vi "fields save field.vi"(8 "error in (no error)":errorcluster, 9 "Post (empty)":T5, 10 "Field Id (\"\")":string, 11 "Connection Refnum":T4) -> (0 "error out":errorcluster, 1 "Field Record":T1={"ixField"=0, "iSequenceOrder"=0, "sxFieldId"="", "sxSequenceId"="", "sDisplayName"="", "sValue"="", "sUnits"="", "nDataType"=enum."timestamp", "nNextItem"=enum."Reset", "fSystem"=FALSE, "fSystemValue"=FALSE, "fRequired"=FALSE, "fSetAtTest"=FALSE, "fTestField"=FALSE, "fDeleted"=FALSE, "fIndexed"=FALSE, "fFreeList"=FALSE}, 3 "Connection Refnum":T4)   [LabVIEW 2011]
uses:
  Addons/internet/utils/keyedarr.llb/Keyed Array.ctl
  SI.LIB/ODBC/SQL Controls/Connection Refnum.ctl
  server/database/Fields/Field Record.ctl
  server/database/Fields/Field DataTypes.ctl
  server/database/Fields/Field NextItem.ctl
  Addons/internet/utils/strutil.llb/Case Matching.ctl
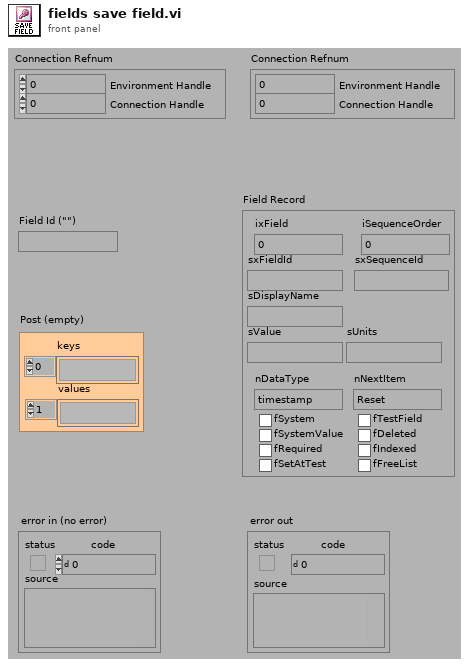
[diagram p1: front panel]
types:
  T1 = typedef "Field Record.ctl" = cluster{"ixField":i32, "iSequenceOrder":i32, "sxFieldId":string, "sxSequenceId":string, "sDisplayName":string, "sValue":string, "sUnits":string, "nDataType":T2, "nNextItem":T3, "fSystem":bool, "fSystemValue":bool, "fRequired":bool, "fSetAtTest":bool, "fTestField":bool, "fDeleted":bool, "fIndexed":bool, "fFreeList":bool}
  T2 = typedef "Field DataTypes.ctl" = enum32{"text", "numeric", "list", "timestamp", "boolean"}
  T3 = typedef "Field NextItem.ctl" = enum32{"Reset", "Retain", "Auto-Increment"}
  T4 = typedef "Connection Refnum.ctl" = cluster{"Environment Handle":i32, "Connection Handle":i32}
  T5 = typedef "Keyed Array.ctl" = cluster{"keys":string[], "values":string[]}
  T6 = typedef "Case Matching.ctl" = enum16{"a != A", "a == A", "system"}
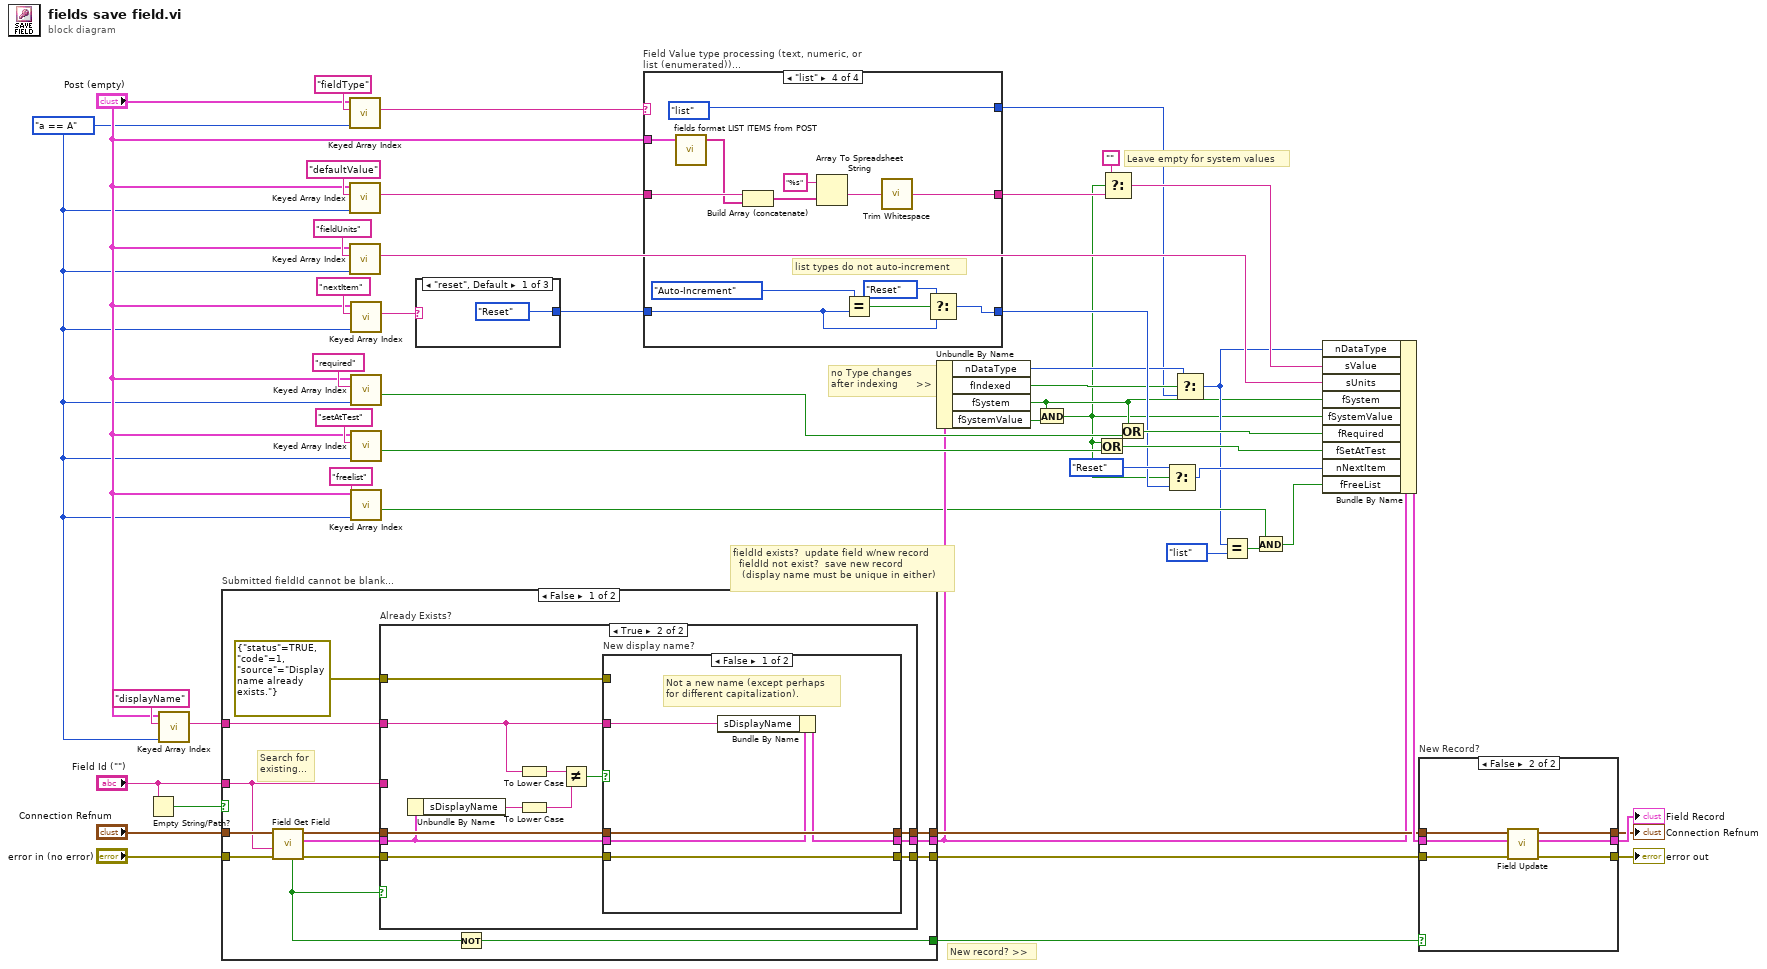
[diagram p0: block diagram]
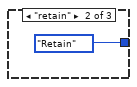
[diagram p2: hidden frame]
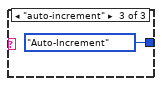
[diagram p3: hidden frame]
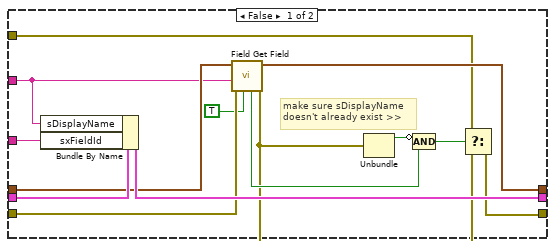
[diagram p4: hidden frame]
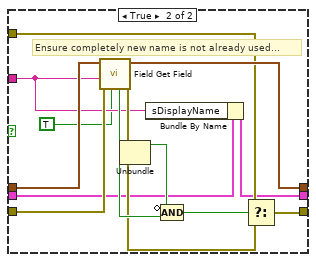
[diagram p5: hidden frame]
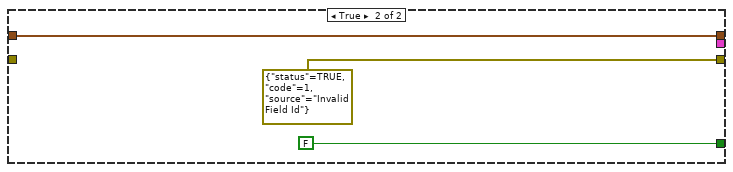
[diagram p6: hidden frame]
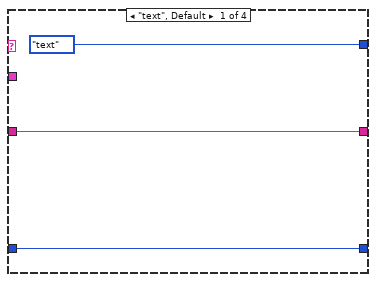
[diagram p7: hidden frame]
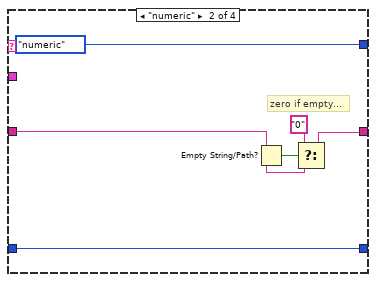
[diagram p8: hidden frame]
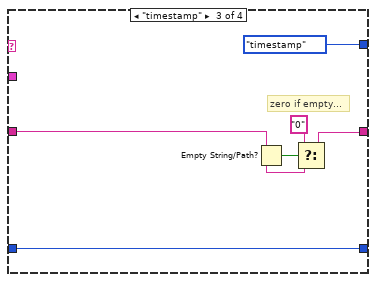
[diagram p9: hidden frame]
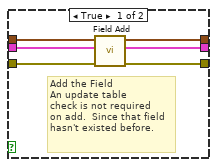
[diagram p10: hidden frame]
diagram:
  w14 = Case_Matching."a == A" ("case matching (sensitive)")
  # "no Type changes\nafter indexing      >>"
  # "Leave empty for system values"
  # "New record? >>"
  # "fieldId exists?  update field w/new record\n  fieldId not exist?  save new record\n   (display name must be unique in either)"
  n1 = Empty String/Path?(string/path="Field Id (\"\")") -> (empty?=w38:bool)
  n2 = call "Keyed Array Index.vi"("case matching (sensitive)"=w14, "key"="displayName", "array in"="Post (empty)") -> ("value"=w27:string)  [unwired: 1 in, 3 out]
  n3 = case "Submitted fieldId cannot be blank..." shown="False" w38 {
    tunnel: "Field Id (\"\")" -> [w52 _]
    tunnel: "Connection Refnum" -> [w62 w108]
    tunnel: "error in (no error)" -> [w61 _]
    tunnel: [w59 FALSE] -> w35
    tunnel: [w55 errorcluster {"status"=TRUE, "code"=1, "source"="Invalid Field Id"} ("error in (no error)")] -> w33
    tunnel: [w54 w108] -> w34
    tunnel: [w53 _] -> w12
    tunnel: w27 -> [w51 _]
    frame False {
      # "Search for\nexisting..."
      n4 = call "Field Get Field.vi"("error in (no error)"=w61, "sFieldId or sDisplayName (\"\")"=w52, "Connection Refnum"=w62) -> ("error out"=w58:errorcluster, "Field"=w56:T1, "Connection Refnum"=w57:T4, "Data Present?"=w60:bool)  [unwired: 2 in, 3 out]
      n5 = case "Already Exists?" shown="True" w60 {
        tunnel: w58 -> [w68 w85]
        tunnel: w57 -> [w70 w86]
        tunnel: w56 -> [w76 w82]
        tunnel: [w67 w84] -> w55
        tunnel: [w69 w83] -> w54
        tunnel: [w74 w81] -> w53
        tunnel: w52 -> [w75 _]
        tunnel: w51 -> [w64 w80]
        tunnel: errorcluster {"status"=TRUE, "code"=1, "source"="Display name already exists."} ("t") -> [w65 w79]
        frame False {
          # "make sure sDisplayName\ndoesn't already exist >>"
          n6 = Bundle By Name(cluster=w76, "sDisplayName"=w64, "sxFieldId"=w75) -> (w74:T1)
          n7 = call "Field Get Field.vi"("by sDisplayName? (f, by sFieldId)"=TRUE, "error in (no error)"=w68, "sFieldId or sDisplayName (\"\")"=w64, "Connection Refnum"=w70) -> ("error out"=w66:errorcluster, "Connection Refnum"=w69:T4, "Data Present?"=w72:bool)  [unwired: 1 in, 4 out]
          n8 = Unbundle(w66) -> ("status"=w73:bool)  [unwired: 2 out]
          n9 = Compound Arithmetic op=AND(invert w73, w72) -> (w71:bool)
          n10 = Select(t=w65, s=w71, f=w66) -> (s? t:f=w67:errorcluster)
        }
        frame True {
          n11 = Unbundle By Name(w82) -> ("sDisplayName"=w88:string)
          n12 = To Lower Case(string=w80) -> (all lower case string=w78:string)
          n13 = To Lower Case(string=w88) -> (all lower case string=w77:string)
          n14 = Not Equal?(x=w78, y=w77) -> (x != y?=w87:bool)
          n15 = case "New display name?" shown="False" w87 {
            tunnel: [w93 w104] -> w83
            tunnel: w86 -> [w93 w106]
            tunnel: [w92 w98] -> w84
            tunnel: w85 -> [w92 w105]
            tunnel: [w90 w95] -> w81
            tunnel: w82 -> [w91 w96]
            tunnel: w80 -> [w89 w97]
            tunnel: w79 -> [_ w99]
            frame False {
              # "Not a new name (except perhaps\nfor different capitalization)."
              n16 = Bundle By Name(cluster=w91, "sDisplayName"=w89) -> (w90:T1)
            }
            frame True {
              # "Ensure completely new name is not already used..."
              n17 = call "Field Get Field.vi"("by sDisplayName? (f, by sFieldId)"=TRUE, "error in (no error)"=w105, "sFieldId or sDisplayName (\"\")"=w97, "Connection Refnum"=w106) -> ("error out"=w100:errorcluster, "Connection Refnum"=w104:T4, "Data Present?"=w102:bool)  [unwired: 1 in, 4 out]
              n18 = Unbundle(w100) -> ("status"=w103:bool)  [unwired: 2 out]
              n19 = Bundle By Name(cluster=w96, "sDisplayName"=w97) -> (w95:T1)
              n20 = Compound Arithmetic op=AND(invert w103, w102) -> (w101:bool)
              n21 = Select(t=w99, s=w101, f=w100) -> (s? t:f=w98:errorcluster)
            }
          }
        }
      }
      n22 = Not(x=w60) -> (.not. x?=w59:bool)
    }
    frame True {
    }
  }
  n23 = call "Keyed Array Index.vi"("case matching (sensitive)"=w14, "key"="fieldType", "array in"="Post (empty)") -> ("value"=w43:string)  [unwired: 1 in, 3 out]
  n24 = call "Keyed Array Index.vi"("case matching (sensitive)"=w14, "key"="defaultValue", "array in"="Post (empty)") -> ("value"=w42:string)  [unwired: 1 in, 3 out]
  n25 = call "Keyed Array Index.vi"("case matching (sensitive)"=w14, "key"="fieldUnits", "array in"="Post (empty)") -> ("value"=w18:string)  [unwired: 1 in, 3 out]
  n26 = call "Keyed Array Index.vi"("case matching (sensitive)"=w14, "key"="nextItem", "array in"="Post (empty)") -> ("value"=w25:string)  [unwired: 1 in, 3 out]
  n27 = call "Keyed Array Index.vi"("case matching (sensitive)"=w14, "key"="required", "array in"="Post (empty)") -> ("valid key"=w31:bool)  [unwired: 1 in, 3 out]
  n28 = call "Keyed Array Index.vi"("case matching (sensitive)"=w14, "key"="setAtTest", "array in"="Post (empty)") -> ("valid key"=w29:bool)  [unwired: 1 in, 3 out]
  n29 = call "Keyed Array Index.vi"("case matching (sensitive)"=w14, "key"="freelist", "array in"="Post (empty)") -> ("valid key"=w10:bool)  [unwired: 1 in, 3 out]
  n30 = case shown="\"reset\", Default" w25 {
    tunnel: [Field_NextItem."Reset" ("nNextItem") Field_NextItem."Retain" ("nNextItem") Field_NextItem."Auto-Increment" ("nNextItem")] -> w24
    frame "reset", Default {
    }
    frame "retain" {
    }
    frame "auto-increment" {
    }
  }
  n31 = case "Field Value type processing (text, numeric, or list (enumerated))..." shown="\"list\"" w43 {
    tunnel: w42 -> [w114 w117 w123 w133]
    tunnel: "Post (empty)" -> [_ _ _ w137]
    tunnel: w24 -> [w115 w121 w127 w138]
    tunnel: [w115 w121 w127 w139] -> w13
    tunnel: [w114 w118 w124 w128] -> w21
    tunnel: [Field_DataTypes."text" ("x") Field_DataTypes."numeric" ("x") Field_DataTypes."timestamp" ("x") Field_DataTypes."list" ("x")] -> w5
    frame "text", Default {
    }
    frame "numeric" {
      # "zero if empty..."
      n32 = Empty String/Path?(string/path=w117) -> (empty?=w120:bool)
      n33 = Select(t="0", s=w120, f=w117) -> (s? t:f=w118:string)
    }
    frame "timestamp" {
      # "zero if empty..."
      n34 = Empty String/Path?(string/path=w123) -> (empty?=w126:bool)
      n35 = Select(t="0", s=w126, f=w123) -> (s? t:f=w124:string)
    }
    frame "list" {
      # "list types do not auto-increment"
      n36 = call "fields format LIST ITEMS from POST.vi"("Post (empty)"=w137) -> ("List Options"=w132:string[])  [unwired: 4 out]
      n37 = Build Array (concatenate)(w133, w132) -> (w131:string[])
      n38 = Array To Spreadsheet String(array=w131, 3:"%s" ("format string")) -> (spreadsheet string=w130:string)  [unwired: 1 out]
      n39 = Equal?(x=Field_NextItem."Auto-Increment" ("nNextItem"), y=w138) -> (x = y?=w140:bool)
      n40 = call <vilib>:"Trim Whitespace.vi"("string"=w130) -> ("trimmed string"=w128:string)  [unwired: 1 in]
      n41 = Select(t=Field_NextItem."Reset" ("nNextItem"), s=w140, f=w138) -> (s? t:f=w139:T3)
    }
  }
  n42 = Unbundle By Name(w12) -> ("nDataType"=w7:T2, "fIndexed"=w6:bool, "fSystem"=w2:bool, "fSystemValue"=w3:bool)
  n43 = And(x=w2, y=w3) -> (x .and. y?=w1:bool)
  n44 = Or(x=w1, y=w29) -> (x .or. y?=w30:bool)
  n45 = Select(t="", s=w1, f=w21) -> (s? t:f=w22:string)
  n46 = Or(x=w2, y=w31) -> (x .or. y?=w32:bool)
  n47 = Select(t=Field_NextItem."Reset" ("nNextItem"), s=w1, f=w13) -> (s? t:f=w19:T3)
  n48 = Select(t=w7, s=w6, f=w5) -> (s? t:f=w4:T2)
  n49 = Equal?(x=w4, y=Field_DataTypes."list" ("x")) -> (x = y?=w11:bool)
  n50 = And(x=w10, y=w11) -> (x .and. y?=w9:bool)
  n51 = Bundle By Name(cluster=w12, "nDataType"=w4, "sValue"=w22, "sUnits"=w18, "fSystem"=w2, "fSystemValue"=w1, "fRequired"=w32, "fSetAtTest"=w30, "nNextItem"=w19, "fFreeList"=w9) -> (w47:T1)
  n52 = case "New Record?" shown="False" w35 {
    tunnel: [w146 w147] -> w49
    tunnel: w34 -> [w145 w151]
    tunnel: w33 -> [w144 w150]
    tunnel: w47 -> [w143 w149]
    tunnel: [w142 w149] -> w48
    tunnel: [w141 w148] -> w28
    frame True {
      # "Add the Field\nAn update table\ncheck is not required\non add.  Since that field\nhasn't existed before."
      n53 = call "Field Add.vi"("error in (no error)"=w144, "Field Record"=w143, "Connection Refnum"=w145) -> ("error out"=w146:errorcluster, "New Field"=w142:T1, "Connection Refnum"=w141:T4)  [unwired: 1 in, 5 out]
    }
    frame False {
      n54 = call "Field Update.vi"("error in (no error)"=w150, "Field Record"=w149, "Connection Refnum"=w151) -> ("error out"=w147:errorcluster, "Connection Refnum"=w148:T4)  [unwired: 7 out]
    }
  }
  "error out" <- w49
  "Connection Refnum" <- w28
  "Field Record" <- w48
